vi "Send YIELD.vi"(8 "error in (no error)":errorcluster, 9 "Yield request":T1={"Invocation Request ID"=0, "Arguments"="[]", "ArgumentsKw"="{}", "Options"="{}"}, 11 "WAMP Client in":refnum<class "WAMP Client.lvclass">) -> (0 "error out":errorcluster, 3 "WAMP Client out":refnum<class "WAMP Client.lvclass">)   [LabVIEW 2020, in "wamplv.lvlib" / "WAMP Client.lvclass"]
uses:
  WAMP Client.lvclass
  TypeDef/YIELD request data.ctl
  WAMP Client.lvclass/WAMP Client.ctl
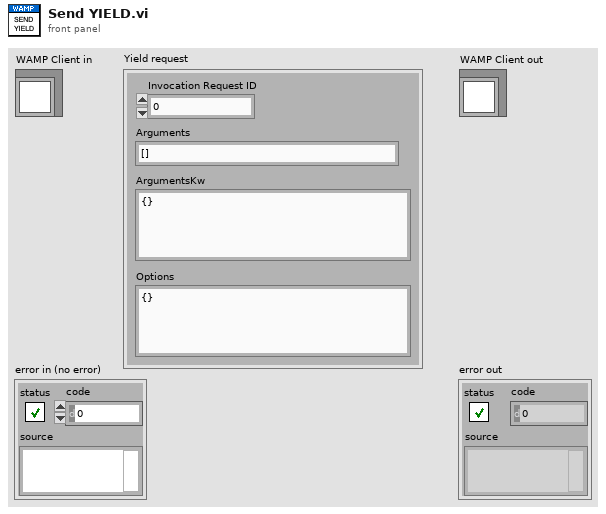
[diagram p1: front panel]
types:
  T1 = typedef "wamplv.lvlib/WAMP Client.lvclass/YIELD request data.ctl" = cluster{"Invocation Request ID":u64, "Arguments":string, "ArgumentsKw":string, "Options":string}
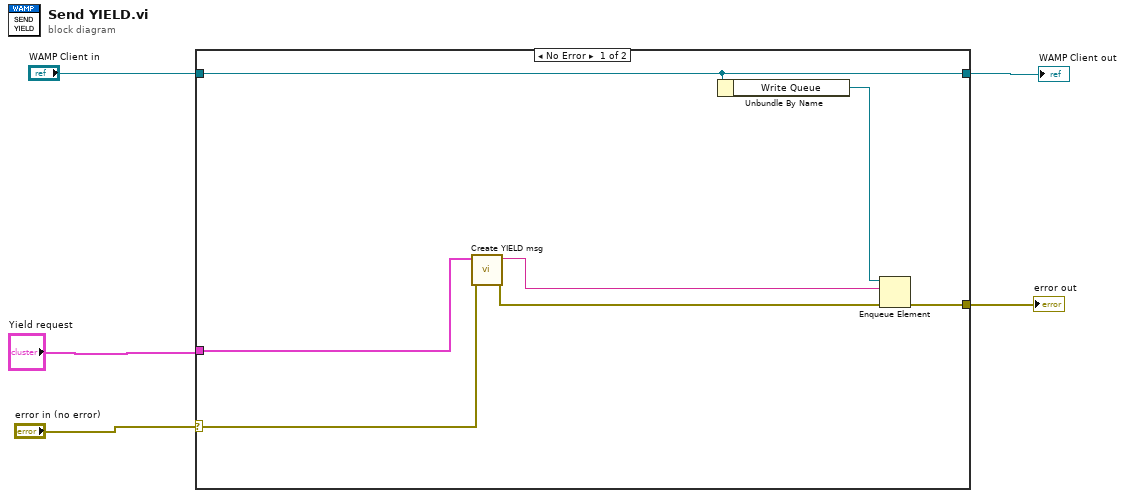
[diagram p0: block diagram]
diagram:
  n1 = case shown="No Error" "error in (no error)" {
    selector: "error in (no error)" -> [w8 w14]
    tunnel: [w12 w14] -> w4
    tunnel: [w7 w13] -> w2
    tunnel: "WAMP Client in" -> [w7 w13]
    tunnel: "Yield request" -> [w6 _]
    frame No Error {
      n2 = call "Create YIELD msg.vi"("error in (no error)"=w8, "Yield request"=w6) -> ("error out"=w10:errorcluster, "String"=w11:string)  [unwired: 8 in]
      n3 = Unbundle By Name(w7) -> ("Write Queue"=w9:refnum<queue>)
      n4 = Enqueue Element(queue=w9, element=w11, error in (no error)=w10) -> (error out=w12:errorcluster)  [unwired: 1 in, 2 out]
    }
    frame Error {
    }
  }
  "error out" <- w4
  "WAMP Client out" <- w2
